vi "ParseDithereImageName.vi"(11 "ImageName":string="<Date Code>_<Project>_DOE123_<Printer Name>_<Printhead #>_Ink Type.bmp") -> (1 "DOE#":string, 2 "InkType":string, 3 "Name Excluding Head and Ink":string)   [LabVIEW 2022 SP3]
uses:
  <vilib>/regexp/Match Regular Expression.xnode
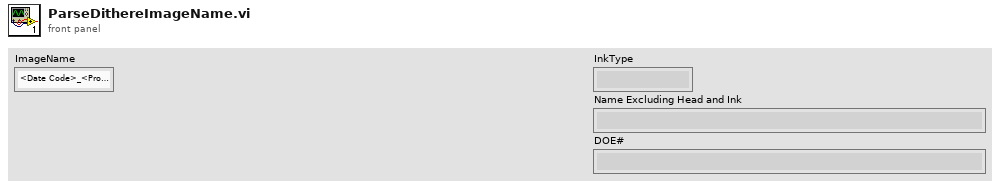
[diagram p1: front panel]
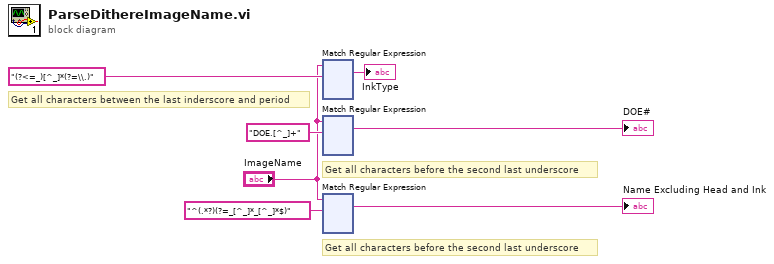
[diagram p0: block diagram]
diagram:
  # "Get all characters before the second last underscore"
  # "Get all characters between the last inderscore and period"
  # "Get all characters before the second last underscore"
  n1 = xnode "Match Regular Expression"("input string"="ImageName", "regular expression"="(?<=_)[^_]*(?=\\.)") -> ("whole match"=→"InkType":string)  [unwired: 4 in, 4 out]
  n2 = xnode "Match Regular Expression"("input string"="ImageName", "regular expression"="DOE.[^_]+") -> ("whole match"=→"DOE#":string)  [unwired: 4 in, 4 out]
  n3 = xnode "Match Regular Expression"("input string"="ImageName", "regular expression"="^(.*?)(?=_[^_]*_[^_]*$)") -> ("whole match"=→"Name Excluding Head and Ink":string)  [unwired: 4 in, 4 out]
